vi "Append Table (string).vi"(7 "Style":T1={"Name"="Default", "Font"={"Name"="Calibri", "Size"=12, "Bold"=FALSE, "Italic"=FALSE, "Underline"=18, "Strike"=FALSE, "Color"=0, "Alignment"=1}} {"Font"."Alignment" items=["LEFT"=1, "CENTER"=2, "RIGHT"=3, "BOTH"=4, "MEDIUM_KASHIDA"=5, "DISTRIBUTE"=6, "NUM_TAB"=7, "HIGH_KASHIDA"=8, "LOW_KASHIDA"=9, "THAI_DISTRIBUTE"=10]; "Font"."Underline" items=["Single"=1, "Words"=2, "Double"=3, "Thick"=4, "Dotted"=5, "DottedHeavy"=6, "Dash"=7, "DashedHeavy"=8, "DashLong"=9, "DashLongHeavy"=10, "DotDash"=11, "DashDotHeavy"=12, "DotDotDash"=13, "DashDotDotHeavy"=14, "Wave"=15, "WavyHeavy"=16, "WavyDouble"=17, "None"=18]}, 8 "error in (no error)":errorcluster, 10 "Table":string[][](array[string]), 11 "Document in":refnum<class "Document.lvclass">) -> (0 "error out":errorcluster, 3 "Document out":refnum<class "Document.lvclass">)   [LabVIEW 2020, in "LabVIEW NPOI.lvlib" / "Document.lvclass"]
doc: "Appends the wire <b>Table</b> as 2D array of strings to the <b>Document</b> as a table."
uses:
  Document.lvclass
  Styles/Style--cluster.ctl
  Styles/Font--cluster.ctl
  Styles/Underline--ring.ctl
  Styles/Alignment--ring.ctl
  Styles/Styles.lvlib
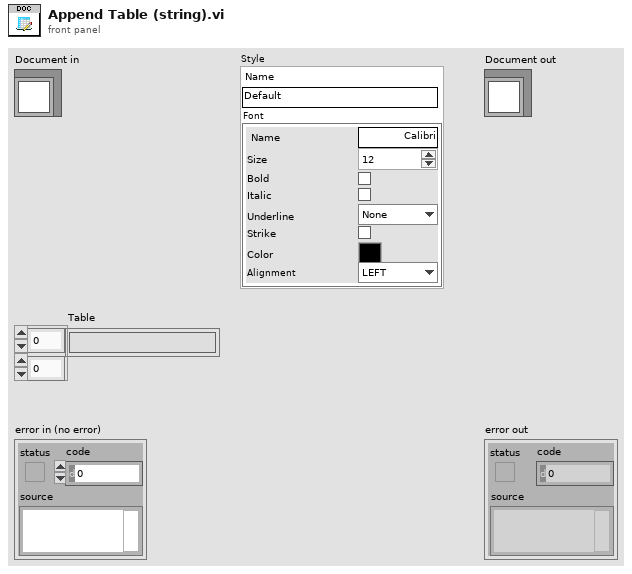
[diagram p1: front panel]
types:
  T1 = typedef "Styles.lvlib/Style--cluster.ctl" = cluster{"Name":string, "Font":T2}
  T2 = typedef "Styles.lvlib/Font--cluster.ctl" = cluster{"Name":string, "Size":i32, "Bold":bool, "Italic":bool, "Underline":T3, "Strike":bool, "Color":u32, "Alignment":T4}
  T3 = typedef "Styles.lvlib/Underline--ring.ctl" = i32
  T4 = typedef "Styles.lvlib/Alignment--ring.ctl" = i32
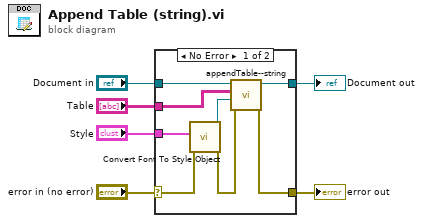
[diagram p0: block diagram]
diagram:
  n1 = case shown="No Error" "error in (no error)" {
    selector: "error in (no error)" -> [w9 w16]
    tunnel: [w11 w16] -> w5
    tunnel: [w13 w15] -> w3
    tunnel: "Document in" -> [w14 w15]
    tunnel: "Table" -> [w12 _]
    tunnel: "Style" -> [w10 _]
    frame No Error {
      n2 = call "Convert Font To Style Object.vi"("error in (no error)"=w9, "Style"=w10) -> ("error out"=w8:errorcluster, "Style Object"=w7:refnum<class "Style.lvclass">)  [unwired: 8 in]
      n3 = call-dynamic "appendTable--string.vi"("error in (no error)"=w8, "Font"=w7, "Table"=w12, "Document in"=w14) -> ("error out"=w11:errorcluster, "Document out"=w13:refnum<class "Document.lvclass">)  [unwired: 6 in]
    }
    frame Error {
    }
  }
  "error out" <- w5
  "Document out" <- w3
